vi "EnvCoverPwrState.vi"(8 "error in (no error)":errorcluster, 11 "PowerState":T1) -> (0 "error out":errorcluster, 3 "PowerState Out":T1)   [LabVIEW 2016]
uses:
  controls/MotorPowerStates.ctl
  controls/RT-Variables.lvlib
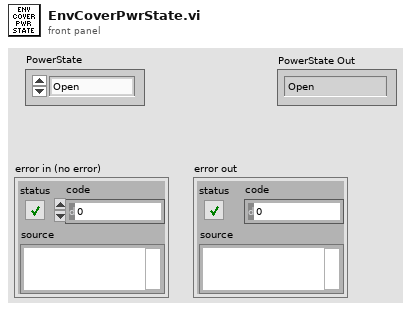
[diagram p1: front panel]
types:
  T1 = typedef "RT-Variables.lvlib/MotorPowerStates.ctl" = enum16{"Open", "Close", "Off"}
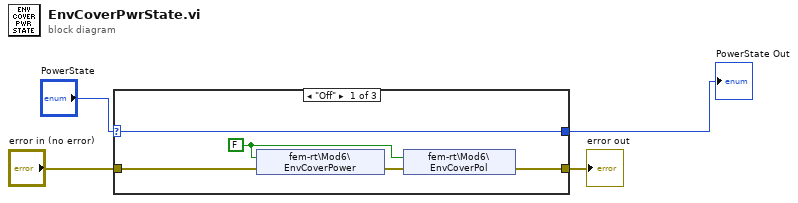
[diagram p0: block diagram]
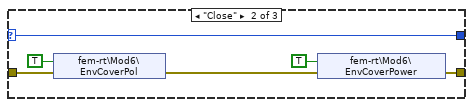
[diagram p2: hidden frame]
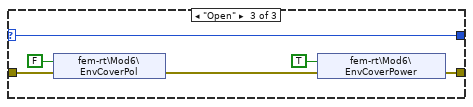
[diagram p3: hidden frame]
diagram:
  n1 = case shown="\"Off\"" "PowerState" {
    selector: "PowerState" -> [w5 w10 w16]
    tunnel: [w7 w12 w18] -> w2
    tunnel: "error in (no error)" -> [w6 w11 w17]
    tunnel: [w5 w10 w16] -> w1
    frame "Off" {
      w9 = FALSE ("EnvCoverPower")
      n2 = shared-variable "fem-rt\\Mod6\\EnvCoverPower"(w9, error in=w6) -> (error out=w8:errorcluster)
      n3 = shared-variable "fem-rt\\Mod6\\EnvCoverPol"(w9, error in=w8) -> (error out=w7:errorcluster)
    }
    frame "Close" {
      n4 = shared-variable "fem-rt\\Mod6\\EnvCoverPol"(TRUE ("EnvCoverPol"), error in=w11) -> (error out=w14:errorcluster)
      n5 = shared-variable "fem-rt\\Mod6\\EnvCoverPower"(TRUE, error in=w14) -> (error out=w12:errorcluster)
    }
    frame "Open" {
      n6 = shared-variable "fem-rt\\Mod6\\EnvCoverPol"(FALSE ("EnvCoverPol"), error in=w17) -> (error out=w20:errorcluster)
      n7 = shared-variable "fem-rt\\Mod6\\EnvCoverPower"(TRUE, error in=w20) -> (error out=w18:errorcluster)
    }
  }
  "error out" <- w2
  "PowerState Out" <- w1
